vi "Change Position.vi"(8 "error in (no error)":errorcluster, 10 "Position Change":i32, 11 "SwipeScrollListbox in":refnum<class "SwipeScrollListbox.lvclass">) -> (0 "error out":errorcluster, 3 "SwipeScrollListbox out":refnum<class "SwipeScrollListbox.lvclass">)   [LabVIEW 2019, in "SwipeScrollListbox.lvclass"]
uses:
  SwipeScrollListbox.lvclass
  C:/Program Files (x86)/National Instruments/LabVIEW 2019/vi.lib/QSI/QControls/QControl Classes/ListBox/ListBox.lvclass
  SwipeScrollListbox.lvclass/SwipeScrollListbox.ctl
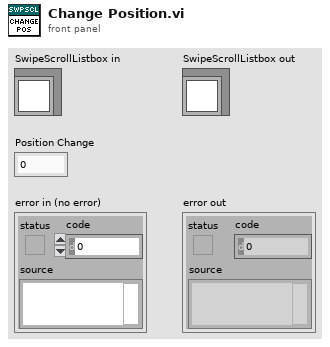
[diagram p1: front panel]
types:
  T1 = typedef "SwipeScrollListbox.lvclass/State Data.ctl" = cluster{"Timeout":i32, "Time":timestamp, "Y":i32, "Slow Distance":i32, "Rate":dbl, "Row Selected":i32}
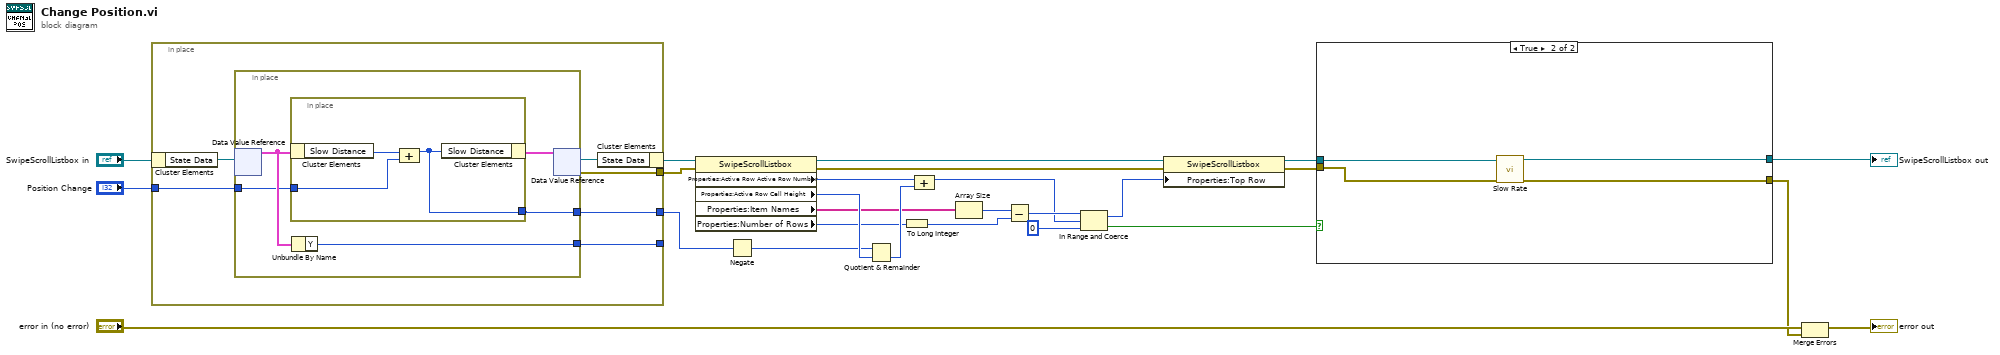
[diagram p0: block diagram]
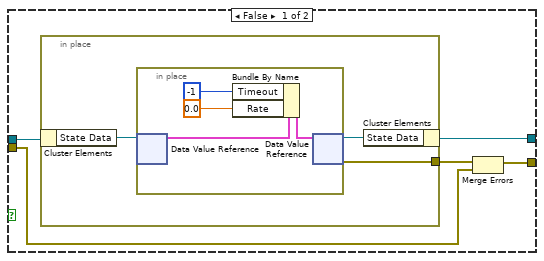
[diagram p2: hidden frame]
diagram:
  n1 = in-place {
    in-place-border: [w30] -> _
    in-place-border: [w29] -> w17
    in-place-border: "Position Change" -> [w28]
    in-place-border: [w27] -> w2
    n2 = in-place-cluster #1("SwipeScrollListbox in") -> ("State Data"=w32:refnum<data-value>)
    n3 = in-place {
      in-place-border: [w37] -> w30
      in-place-border: w28 -> [w35]
      in-place-border: [w34] -> w27
      n4 = in-place-dvr #2(w32) -> (w36:T1)  [unwired: 1 out]
      n5 = in-place {
        in-place-border: w35 -> [w39]
        in-place-border: [w38] -> w34
        n6 = in-place-cluster #3(w36) -> ("Slow Distance"=w40:i32)
        n7 = Compound Arithmetic op=ADD(w40, w39) -> (w38:i32)
        n8 = in-place-cluster #3("Slow Distance"=w38) -> (w33:T1)
      }
      n9 = Unbundle By Name(w36) -> ("Y"=w37:i32)
      n10 = in-place-dvr #2(w33) -> (w31:refnum<data-value>, w29:errorcluster)
    }
    n11 = in-place-cluster #1("State Data"=w31) -> (w19:refnum<class "SwipeScrollListbox.lvclass">)
  }
  n12 = property on="Property Node" class="SwipeScrollListbox"(reference=w19, error in=w17) -> (reference out=w15:refnum<class "SwipeScrollListbox.lvclass">, error out=w21:errorcluster, "Properties:Active Row Active Row Number"=w23:i32, "Properties:Active Row Cell Height"=w20:i32, "Properties:Item Names"=w16:string[], "Properties:Number of Rows"=w13:u32)
  n13 = Negate(x=w2) -> (-x=w1:i32)
  n14 = Quotient & Remainder(x=w1, y=w20) -> (floor(x/y)=w22:i32)  [unwired: 1 out]
  n15 = To Long Integer(number=w13) -> (32bit integer=w11:i32)
  n16 = Compound Arithmetic op=ADD(w23, w22) -> (w9:i32)
  n17 = Array Size(array=w16) -> (size(s)=w14:i32)
  n18 = Subtract(x=w14, y=w11) -> (x-y=w12:i32)
  n19 = In Range and Coerce(upper limit=w12, x=w9, lower limit=0) -> (coerced(x)=w8:i32, In Range?=w7:bool)
  n20 = property on="Property Node" class="SwipeScrollListbox"(reference=w15, error in=w21, "Properties:Top Row"=w8) -> (reference out=w6:refnum<class "SwipeScrollListbox.lvclass">, error out=w5:errorcluster)
  n21 = case shown="True" w7 {
    tunnel: [w45 w56] -> w4
    tunnel: w5 -> [w42 w54]
    tunnel: [w43 w53] -> w3
    tunnel: w6 -> [w41 w55]
    frame False {
      n22 = in-place {
        in-place-border: [w46] -> w44
        n23 = in-place-cluster #4(w41) -> ("State Data"=w48:refnum<data-value>)
        n24 = in-place {
          n25 = in-place-dvr #5(w48) -> (w50:T1)  [unwired: 1 out]
          n26 = Bundle By Name(cluster=w50, "Timeout"=-1, "Rate"=0.0) -> (w49:T1)
          n27 = in-place-dvr #5(w49) -> (w47:refnum<data-value>, w46:errorcluster)
        }
        n28 = in-place-cluster #4("State Data"=w47) -> (w45:refnum<class "SwipeScrollListbox.lvclass">)
      }
      n29 = Merge Errors(w44, w42) -> (w43:errorcluster)
    }
    frame True {
      n30 = call "Slow Rate.vi"("error in (no error)"=w54, "SwipeScrollListbox in"=w55) -> ("error out"=w53:errorcluster, "SwipeScrollListbox out"=w56:refnum<class "SwipeScrollListbox.lvclass">)  [unwired: 8 in]
    }
  }
  "SwipeScrollListbox out" <- w4
  n31 = Merge Errors("error in (no error)", w3) -> (→"error out":errorcluster)
